vi "Send CAN Message.vi"(7 "Number of Retries":i32=5, 8 "error in (no error)":errorcluster, 10 "payload":u8[](array[numeric]), 11 "Gas In":refnum<class "PAS.lvclass">) -> (0 "error out":errorcluster, 2 "Reply":T1[](array[typedef]) {"payload" format="%x"; "timestamp" format="%<%.7X\n%x>T"; "type" items=["CAN Data"=0, "CAN Remote"=1, "CAN Bus Error"=2, "J1939 Data"=192, "Delay"=224, "Log Trigger"=225, "Start Trigger"=226]; "identifier" format="%x"}, 3 "Gas Out":refnum<class "PAS.lvclass">)   [LabVIEW 2015, in "PAS.lvclass"]
doc: "This VI sends a CAN frame to a device through the CAN network and recieves a frame back as a response. This VI is to facilitate the communication ONLY. The custom error handling of every message must be handled in the owning VI"
uses:
  PAS.lvclass
  <vilib>/xnet/xnet.llb/XNET Frame CAN.ctl
  <vilib>/xnet/xnet.llb/XNET Frame Type CAN.ctl
  PAS.lvclass/PAS.ctl
  <vilib>/xnet/xnet.llb/XNET Write (Frame CAN).vi
  <vilib>/xnet/xnet.llb/XNET Read (Frame CAN).vi
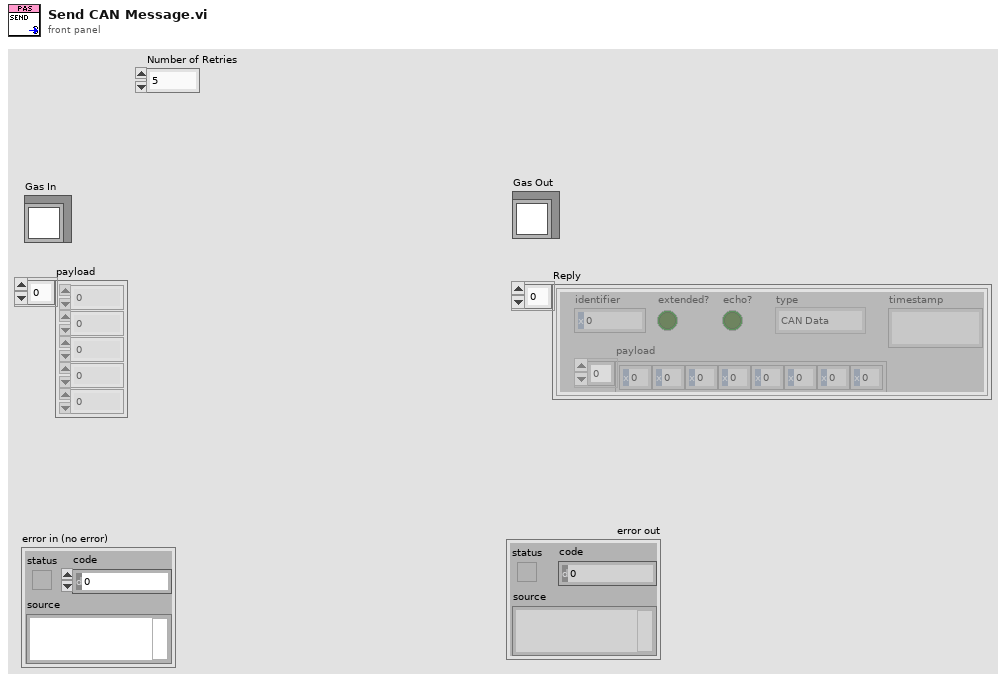
[diagram p1: front panel]
types:
  T1 = typedef "XNET Frame CAN.ctl" = cluster{"timestamp":timestamp, "payload":u8[], "identifier":u32, "type":T2, "extended?":bool, "echo?":bool}
  T2 = typedef "XNET Frame Type CAN.ctl" = u8
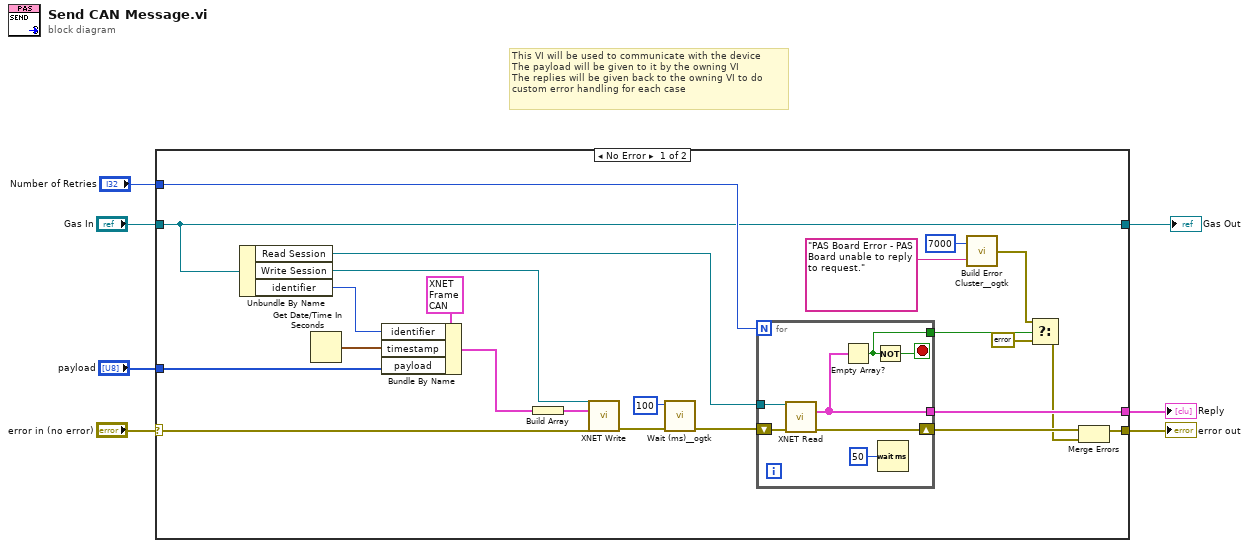
[diagram p0: block diagram]
diagram:
  # "This VI will be used to communicate with the device\nThe payload will be given to it by the owning VI\nThe replies will be given back to the owning VI to do\ncustom error handling for each case"
  n1 = case shown="No Error" "error in (no error)" {
    selector: "error in (no error)" -> [w25 w39]
    tunnel: [w8 w39] -> w7
    tunnel: "Gas In" -> [w16 w38]
    tunnel: [w16 w38] -> w1
    tunnel: "payload" -> [w21 _]
    tunnel: [w18 _] -> w4
    tunnel: "Number of Retries" -> [w17 _]
    frame No Error {
      n2 = Unbundle By Name(w16) -> ("Read Session"=w27:refnum<k21>, "Write Session"=w30:refnum<k21>, "identifier"=w23:u32)
      n3 = Get Date/Time In Seconds() -> (seconds since 1Jan1904=w22:timestamp)
      n4 = Bundle By Name(cluster=T1 {"timestamp"=timestamp(0 s since 1904-01-01), "payload"=[], "identifier"=0, "type"=0, "extended?"=FALSE, "echo?"=FALSE} ("CAN frame"), "identifier"=w23, "timestamp"=w22, "payload"=w21) -> (w20:T1)
      n5 = Build Array(w20) -> (w19:T1[])
      n6 = call-poly <vilib>:"XNET Write.vi"("session in"=w30, "data"=w19, "error in (no error)"=w25) -> ("error out"=w29:errorcluster)  [unwired: 12 out]
      n7 = call <userlib>:"Wait (ms)__ogtk.vi"("error in (no error)"=w29, "milliseconds to wait"=u32 100) -> ("error out"=w26:errorcluster)  [unwired: 8 in, 1 out]
      n8 = for {
        N: w17 -> [_]
        tunnel: w27 -> [w37]
        shift-right: [w35] -> w10
        shift-left: w26 -> [w36]
        tunnel: [w33] -> w18
        tunnel: [w31] -> w15
        stop <- w34 stop-if-true
        n9 = call-poly <vilib>:"XNET Read.vi"("session in"=w37, "error in (no error)"=w36) -> ("data"=w33:T1[], "error out"=w35:errorcluster)  [unwired: 12 out]
        n10 = Empty Array?(array=w33) -> (empty?=w31:bool)
        n11 = Not(x=w31) -> (.not. x?=w34:bool)
        n12 = Wait (ms)(milliseconds to wait=u32 50) -> ()  [unwired: 1 out]
      }
      n13 = call <userlib>:"Build Error Cluster__ogtk.vi"("String to Prepend to source (\"\")"="PAS Board Error - PAS Board unable to reply to request." ("string"), "code"=7000) -> ("error out"=w12:errorcluster)
      n14 = Select(t=w12, s=w15, f=errorcluster {"status"=FALSE, "code"=0, "source"=""}) -> (s? t:f=w9:errorcluster)
      n15 = Merge Errors(w10, w9) -> (w8:errorcluster)
    }
    frame Error {
    }
  }
  "error out" <- w7
  "Reply" <- w4
  "Gas Out" <- w1
